vi "MainConfigUI.vi"(10 "Plugin info":T3, 11 "Input Data":T1={"BasePath"=path "C:/CustomDashboard/MainConfig", "CommunicationData"={"TargetFilePath"="/media/sda1", "ConnectionData"={"host"="roborio-223-frc.local", "user"="lvuser", "password"="", "port"=22}}}) -> ()   [LabVIEW 2015]
uses:
  General/CorePluginInfo.ctl
  ConfigXML/typedefs/MotorControl.ctl
  ConfigXML/typedefs/EncoderControl.ctl
  ConfigXML/typedefs/PIDControl.ctl
  ConfigXML/typedefs/SetpointArrControl.ctl
  ConfigXML/typedefs/ConfigXMLInputData.ctl
  General/RemoteFiles/connectionData.ctl
  ConfigXML/src/ConfigXMLControl.ctl
panel:
  in  "ViewConfigText":bool
  out "Config Currently on Target":string
  out "windowName":string
  in  "ViewCfgOnBot":bool
  in  "ULConfigtoRIO":bool
  in  "LoadConfig":bool
  in  "SaveConfig":bool
  in  "Tab Control":T4(tab)
  in  "IntakeLift":T9
  in  "ChooChoo":T9
  in  "IntakeWheels":cluster{"motor":T5}
  in  "DriveTrain":T10
  in  "General":T11
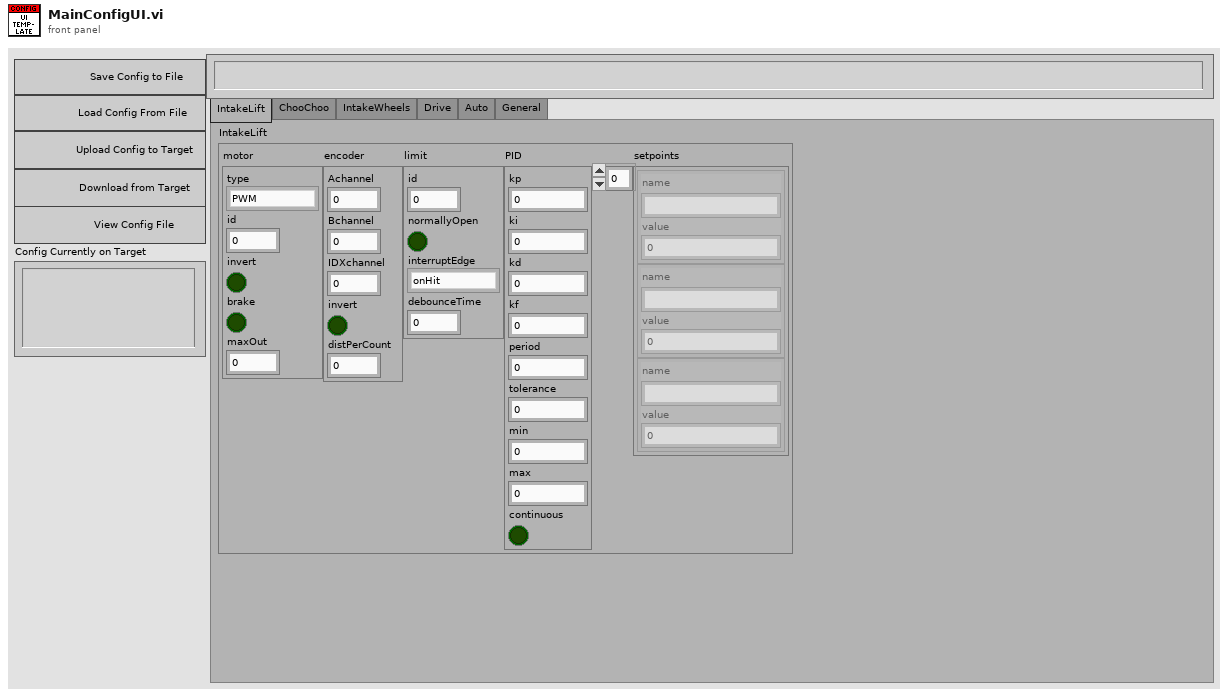
[diagram p1: front panel]
types:
  T1 = typedef "ConfigXMLInputData.ctl" = cluster{"BasePath":path, "CommunicationData":cluster{"TargetFilePath":string, "ConnectionData":T2}}
  T2 = typedef "connectionData.ctl" = cluster{"host":string, "user":string, "password":string, "port":u16}
  T3 = typedef "CorePluginInfo.ctl" = cluster{"Notifiers":cluster{"Robot IP Notifier":refnum<notifier>, "Window Mode Notifier":refnum<notifier>, "Stop Notifier":refnum<notifier>}}
  T4 = enum32{"IntakeLift", "ChooChoo", "IntakeWheels", "Drive", "Auto", "General"}
  T5 = typedef "MotorControl.ctl" = cluster{"type":enum16{"PWM", "CANTalon"}, "id":i32, "invert":bool, "brake":bool, "maxOut":dbl}
  T6 = typedef "EncoderControl.ctl" = cluster{"Achannel":i32, "Bchannel":i32, "IDXchannel":i32, "invert":bool, "distPerCount":dbl}
  T7 = typedef "PIDControl.ctl" = cluster{"kp":dbl, "ki":dbl, "kd":dbl, "kf":dbl, "period":dbl, "tolerance":dbl, "min":dbl, "max":dbl, "continuous":bool}
  T8 = typedef "SetpointArrControl.ctl" = cluster{"name":string, "value":dbl}[]
  T9 = cluster{"motor":T5, "encoder":T6, "limit":cluster{"id":i32, "normallyOpen":bool, "interruptEdge":enum16{"onHit", "onRelease", "both"}, "debounceTime":dbl}, "PID":T7, "setpoints":T8}
  T10 = cluster{"leftSide":cluster{"Motors":T5[], "encoder":T6, "PID":T7}, "rightSide":cluster{"Motors":T5[], "encoder":T6, "PID":T7}, "distancePID":T7, "anglePID":T7, "maxOut":dbl, "fineAdj":dbl, "wheelBaseWidth":dbl}
  T11 = cluster{"flashlight":cluster{"holdTime":dbl, "relayPort":i32}, "zeroLiftAndCCDelay":dbl}
  T12 = typedef "ConfigXMLControl.ctl" = cluster{"ViewCfgOnTarget":refnum<vi>, "ULConfigtoTarget":refnum<vi>, "TabControl":refnum<vi>, "ConfigOnTarget":refnum<vi>, "LoadConfig":refnum<vi>, "SaveConfig":refnum<vi>, "BaseDirectory":path, "TargetFilePath":string, "ViewConfigText":refnum<vi>, "Plugin Info":T3}
  T13 = cluster{"TargetFilePath":string, "ConnectionData":T2}
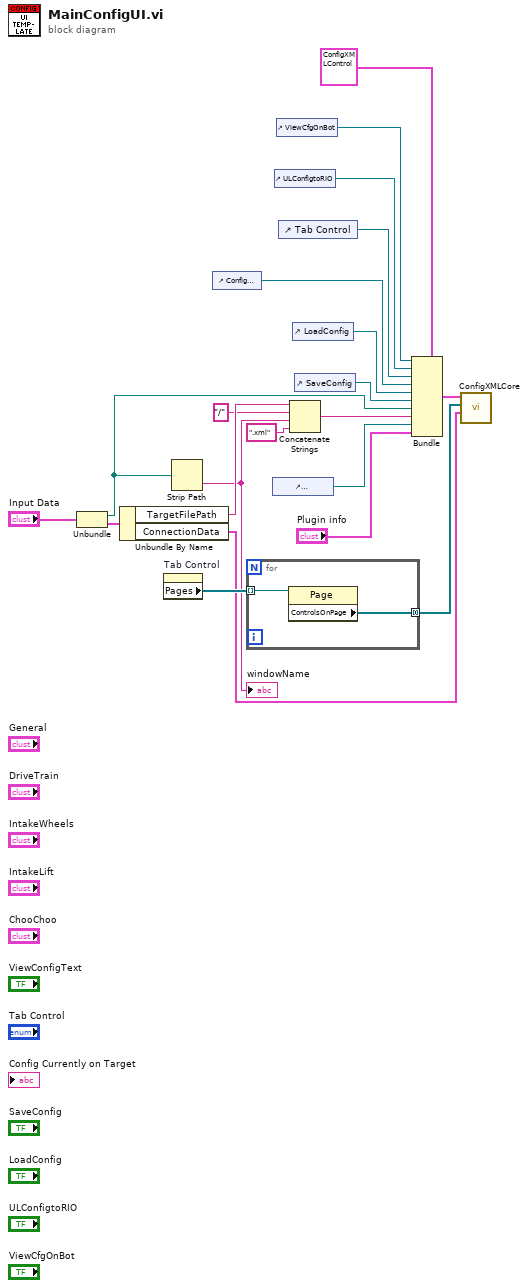
[diagram p0: block diagram]
diagram:
  n1 = Unbundle("Input Data") -> ("BasePath"=w2:path, "CommunicationData"=w1:T13)
  n2 = Unbundle By Name(w1) -> ("TargetFilePath"=w10:string, "ConnectionData"=w11:T2)
  n3 = property on="Tab Control" class="TabCtl (strict)"() -> ("Pages"=w21:refnum<vi>[])  [unwired: 2 in, 2 out]
  n4 = Strip Path(path=w2) -> (name=w8:string)  [unwired: 1 out]
  "windowName" <- w8
  n5 = control-ref of="Config Currently on Target"() -> (w13:refnum<vi>)
  n6 = for {
    tunnel: w21 -> [w23] mode=indexing
    tunnel: [w22] -> w14 mode=concatenating
    n7 = property class="Page"(reference=w23) -> ("ControlsOnPage"=w22:refnum<vi>[])  [unwired: 1 in, 2 out]
  }
  n8 = control-ref of="ViewConfigText"() -> (w5:refnum<vi>)
  n9 = control-ref of="ULConfigtoRIO"() -> (w19:refnum<vi>)
  n10 = control-ref of="ViewCfgOnBot"() -> (w20:refnum<vi>)
  n11 = control-ref of="Tab Control"() -> (w12:refnum<vi>)
  n12 = Concatenate Strings(w10, "/" ("string"), w8, ".xml" ("string")) -> (w6:string)
  n13 = control-ref of="LoadConfig"() -> (w18:refnum<vi>)
  n14 = control-ref of="SaveConfig"() -> (w17:refnum<vi>)
  n15 = Bundle(cluster=T12 {"ViewCfgOnTarget"=refnum, "ULConfigtoTarget"=refnum, "TabControl"=refnum, "ConfigOnTarget"=refnum, "LoadConfig"=refnum, "SaveConfig"=refnum, "BaseDirectory"=path "", "TargetFilePath"="", "ViewConfigText"=refnum, "Plugin Info"={"Notifiers"={"Robot IP Notifier"=refnum, "Window Mode Notifier"=refnum, "Stop Notifier"=refnum}}} ("output cluster"), "ViewCfgOnTarget"=w20, "ULConfigtoTarget"=w19, "TabControl"=w12, "ConfigOnTarget"=w13, "LoadConfig"=w18, "SaveConfig"=w17, "BaseDirectory"=w2, "TargetFilePath"=w6, "ViewConfigText"=w5, "Plugin Info"="Plugin info") -> (w15:T12)
  n16 = call "ConfigXMLCore.vi"("ConnectionData"=w11, "controlsToSave"=w14, "ConfigXMLControl"=w15) -> ()  [unwired: 9 in]
